vi "Check for stable temperature.vi"(7 "Actual Temperature":sgl, 10 "Set Temperature":sgl) -> (0 "Temperature in Range":bool, 3 "Temperature Stable":bool)   [LabVIEW 2016]
uses:
  <vilib>/Analysis/baseanly.llb/Mean (DBL).vi
  Miscellaneous/Globals.vi
  <vilib>/Analysis/NI_AALBase.lvlib
panel:
  out "XY Graph":cluster{dbl[], dbl[]}(graph)
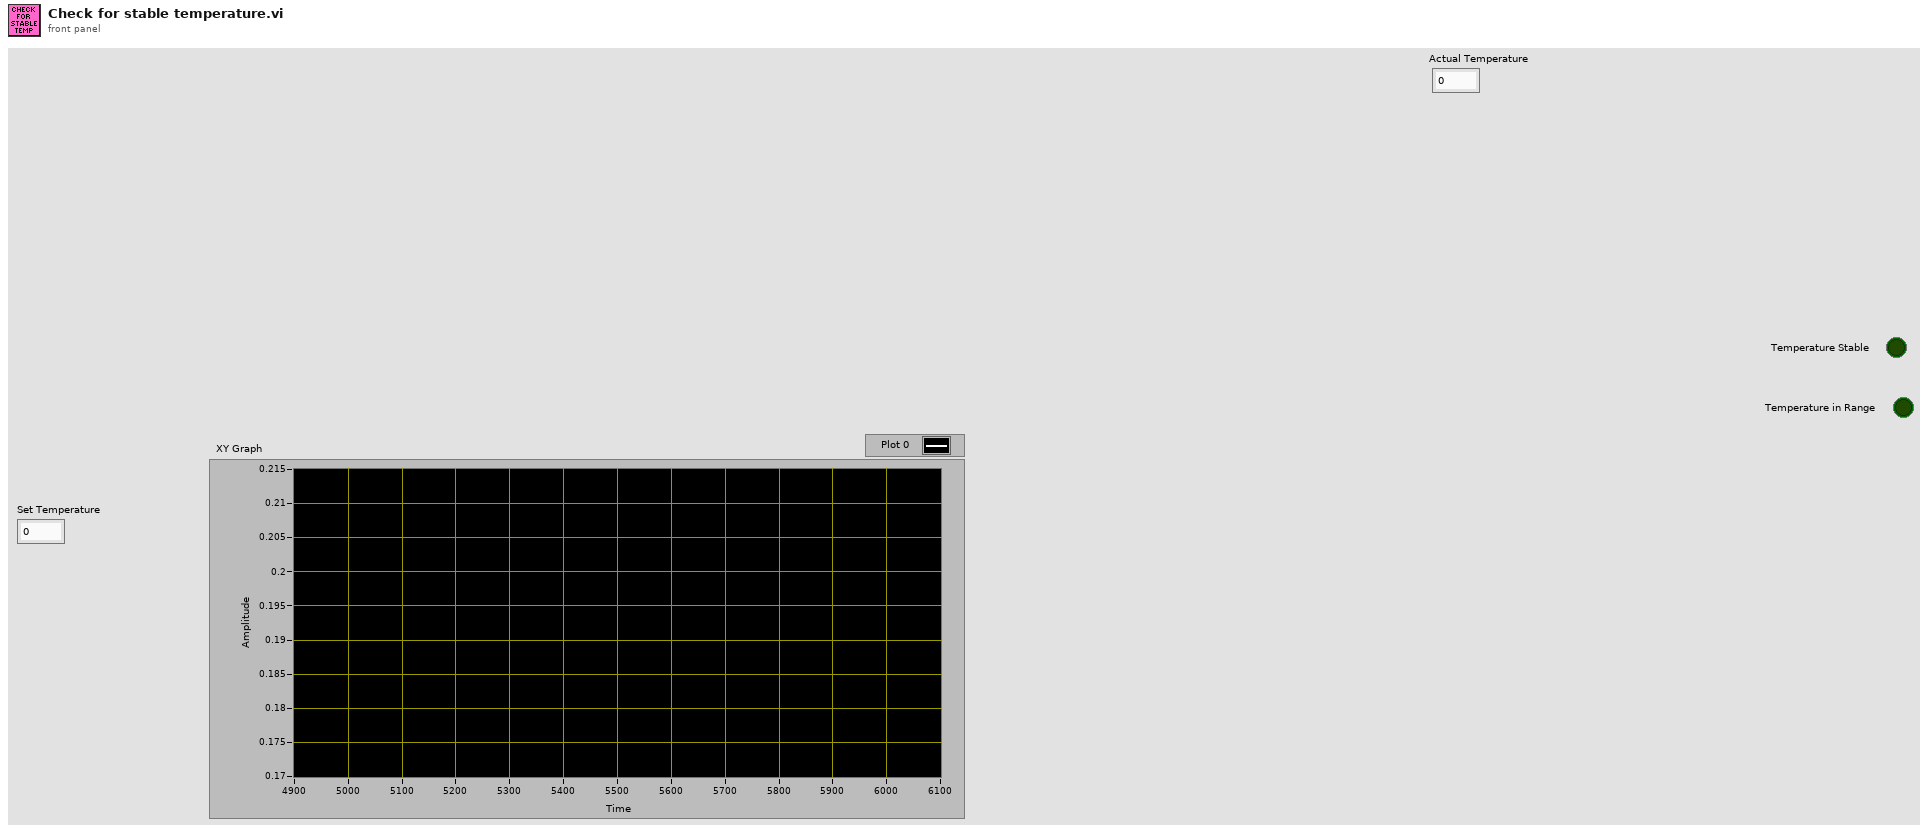
[diagram p1: front panel]
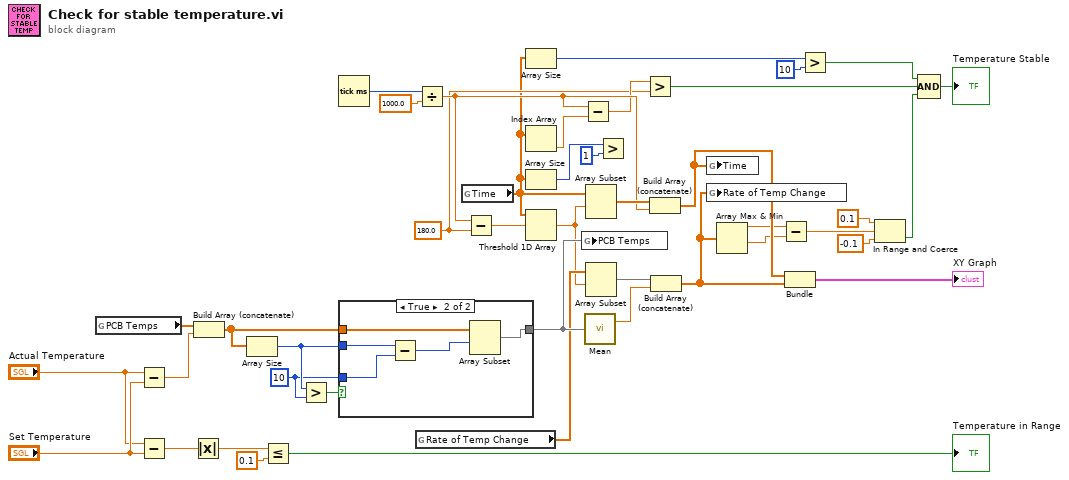
[diagram p0: block diagram]
diagram:
  w10 = 180.0 ("y")
  w33 = 10 ("y")
  n1 = global read "Globals.vi" "PCB Temps"() -> (w37:dbl[])
  n2 = Subtract(x="Actual Temperature", y="Set Temperature") -> (x-y=w38:sgl)
  n3 = Subtract(x="Actual Temperature", y="Set Temperature") -> (x-y=w41:sgl)
  n4 = Absolute Value(x=w41) -> (abs(x)=w40:sgl)
  n5 = Build Array (concatenate)(w37, w38) -> (w35:dbl[])
  n6 = Array Size(array=w35) -> (size(s)=w34:i32)
  n7 = Less Or Equal?(x=w40, y=0.1) -> (x <= y?=→"Temperature in Range":bool)
  n8 = Greater?(x=w34, y=w33) -> (0:w36:bool)
  n9 = Tick Count (ms)() -> (millisecond timer value=w31:u32)
  n10 = case shown="True" w36 {
    tunnel: w35 -> [w43 w48]
    tunnel: w34 -> [_ w47]
    tunnel: w33 -> [_ w46]
    tunnel: [w43 w44] -> w32
    frame False {
    }
    frame True {
      n11 = Subtract(x=w47, y=w46) -> (x-y=w45:i32)
      n12 = Array Subset(array=w48, index=w45) -> (w44:dbl[])  [unwired: 1 in]
    }
  }
  n13 = global read "Globals.vi" "Rate of Temp Change"() -> (w27:dbl[])
  n14 = Divide(x=w31, y=1000.0) -> (x/y=w13:dbl)
  n15 = global read "Globals.vi" "Time"() -> (w7:dbl[])
  n16 = Subtract(x=w13, y=w10) -> (x-y=w29:dbl)
  n17 = Array Size(array=w7) -> (size(s)=w6:i32)
  n18 = Index Array(array=w7) -> (element=w12:dbl)  [unwired: 1 in]
  n19 = Array Size(array=w7) -> (size(s)=w23:i32)
  n20 = Threshold 1D Array(2:w29, 3:w7) -> (0:w25:dbl)  [unwired: 1 in]
  n21 = global write "Globals.vi" "PCB Temps"(w32) -> ()
  n22 = Subtract(x=w13, y=w12) -> (x-y=w11:dbl)
  n23 = call-poly <vilib>:"Mean.vi"("X"=w32) -> ("mean"=w21:dbl)  [unwired: 1 out]
  n24 = Array Subset(array=w7, index=w25) -> (w24:dbl[])  [unwired: 1 in]
  n25 = Array Subset(array=w27, index=w25) -> (w26:dbl[])  [unwired: 1 in]
  n26 = Greater?(x=w23, y=1) -> ()  [unwired: 1 out]
  n27 = Greater?(x=w11, y=w10) -> (0:w9:bool)
  n28 = Build Array (concatenate)(w24, w13) -> (w28:dbl[])
  n29 = Build Array (concatenate)(w26, w21) -> (w19:dbl[])
  n30 = global write "Globals.vi" "Time"(w28) -> ()
  n31 = global write "Globals.vi" "Rate of Temp Change"(w19) -> ()
  n32 = Array Max & Min(array=w19) -> (max value=w18:dbl, min value=w17:dbl)  [unwired: 2 out]
  n33 = Subtract(x=w18, y=w17) -> (x-y=w16:dbl)
  n34 = Bundle(w28, w19) -> (→"XY Graph":cluster{dbl[], dbl[]})  [unwired: 1 in]
  n35 = Greater?(x=w6, y=10) -> (0:w4:bool)
  n36 = In Range and Coerce(upper limit=0.1, x=w16, lower limit=-0.1) -> (In Range?=w8:bool)  [unwired: 1 out]
  n37 = Compound Arithmetic op=AND(w4, w9, w8) -> (→"Temperature Stable":bool)
